vi "Write Temperature status.vi"(8 "error in (no error)":errorcluster, 10 "Acquisition status":T1, 11 "Temp params in":refnum<class "CV-Temperature.lvclass">) -> (0 "error out":errorcluster, 3 "Temp params out":refnum<class "CV-Temperature.lvclass">)   [LabVIEW 2013, in "CameraVision.lvlib" / "CV-Temperature.lvclass"]
uses:
  CV-Temperature.lvclass
  UI/Module-states.ctl
  CV-Temperature.lvclass/CV-Temperature.ctl
  UI/CV-UI.lvclass
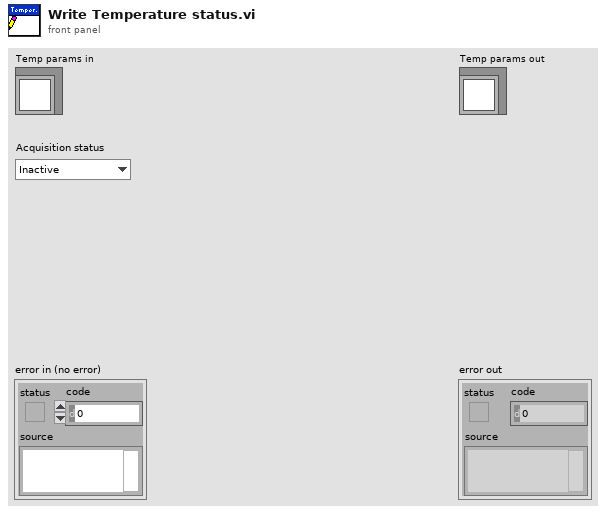
[diagram p1: front panel]
types:
  T1 = typedef "CameraVision.lvlib/CV-UI.lvclass/Module-states.ctl" = enum16{"Inactive", "Active", "Data-loss", "Error", "Simulation", "Synchronizing", "Initialized", "Released"}
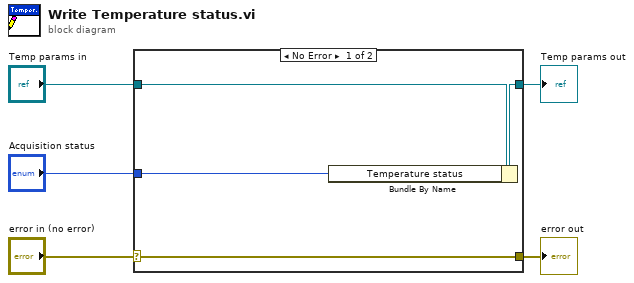
[diagram p0: block diagram]
diagram:
  n1 = case shown="No Error" "error in (no error)" {
    selector: "error in (no error)" -> [w9 w10]
    tunnel: [w9 w10] -> w4
    tunnel: [w7 w11] -> w2
    tunnel: "Temp params in" -> [w8 w11]
    tunnel: "Acquisition status" -> [w6 _]
    frame No Error {
      n2 = Bundle By Name(cluster=w8, "Temperature status"=w6) -> (w7:refnum<class "CV-Temperature.lvclass">)
    }
    frame Error {
    }
  }
  "error out" <- w4
  "Temp params out" <- w2
